vi "Marcus_3dscene.vi"() -> ()   [LabVIEW 2020]
uses:
  <vilib>/picture/3D Picture Control/Object/Create Object (name).vi
  <vilib>/picture/3D Picture Control/NI_3D Picture Control.lvlib
panel:
  in  "Dial 6":dbl(knob) scale=0.0..270.0
  in  "Dial 5":dbl(knob) scale=0.0..270.0
  in  "Dial 4":dbl(knob) scale=0.0..270.0
  in  "Dial 3":dbl(knob) scale=0.0..270.0
  in  "Dial 2":dbl(knob) scale=0.0..270.0
  in  "Dial":dbl(knob) scale=0.0..270.0
  in  "Stop":bool
  out "3D Picture":refnum<vi>(3d-picture)
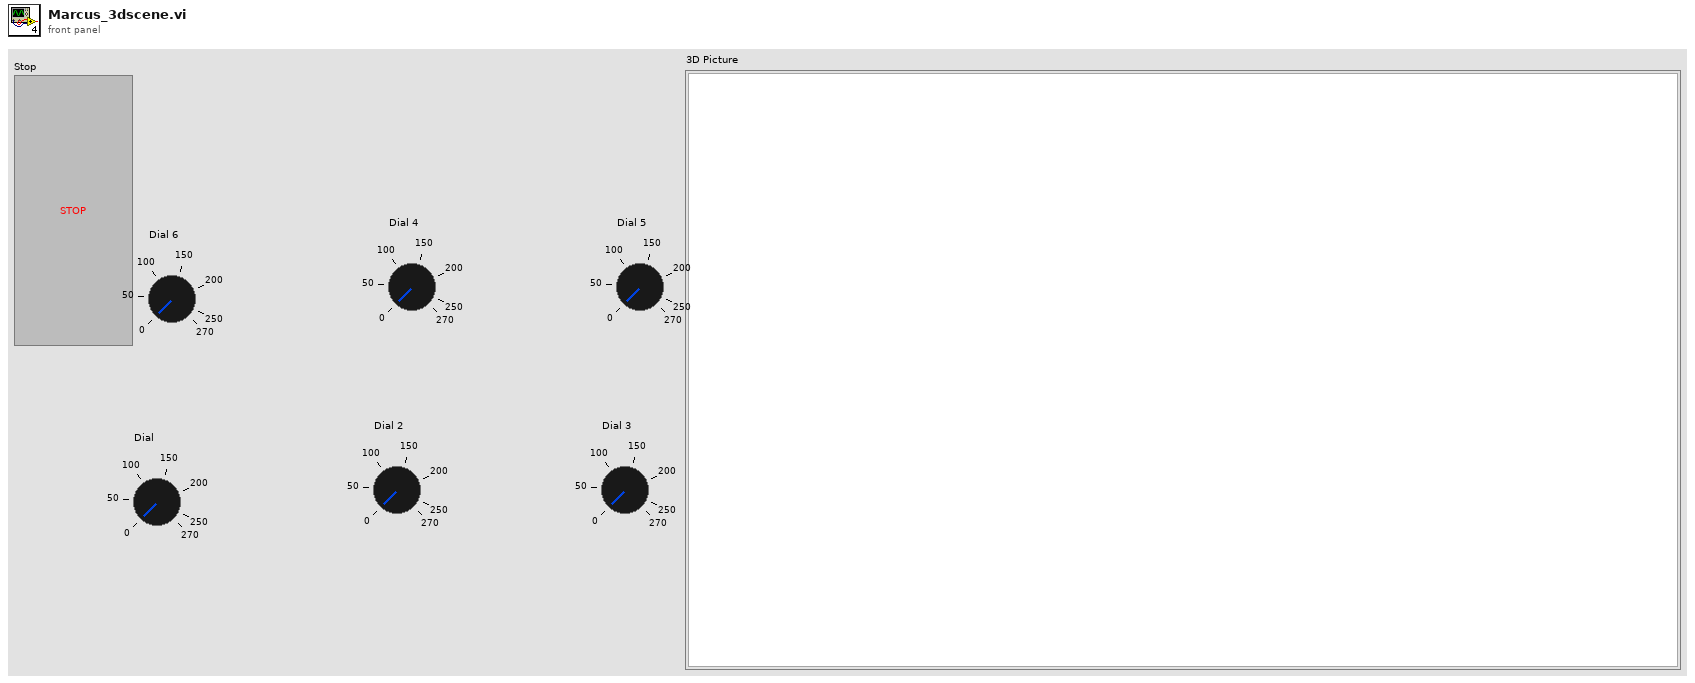
[diagram p1: front panel]
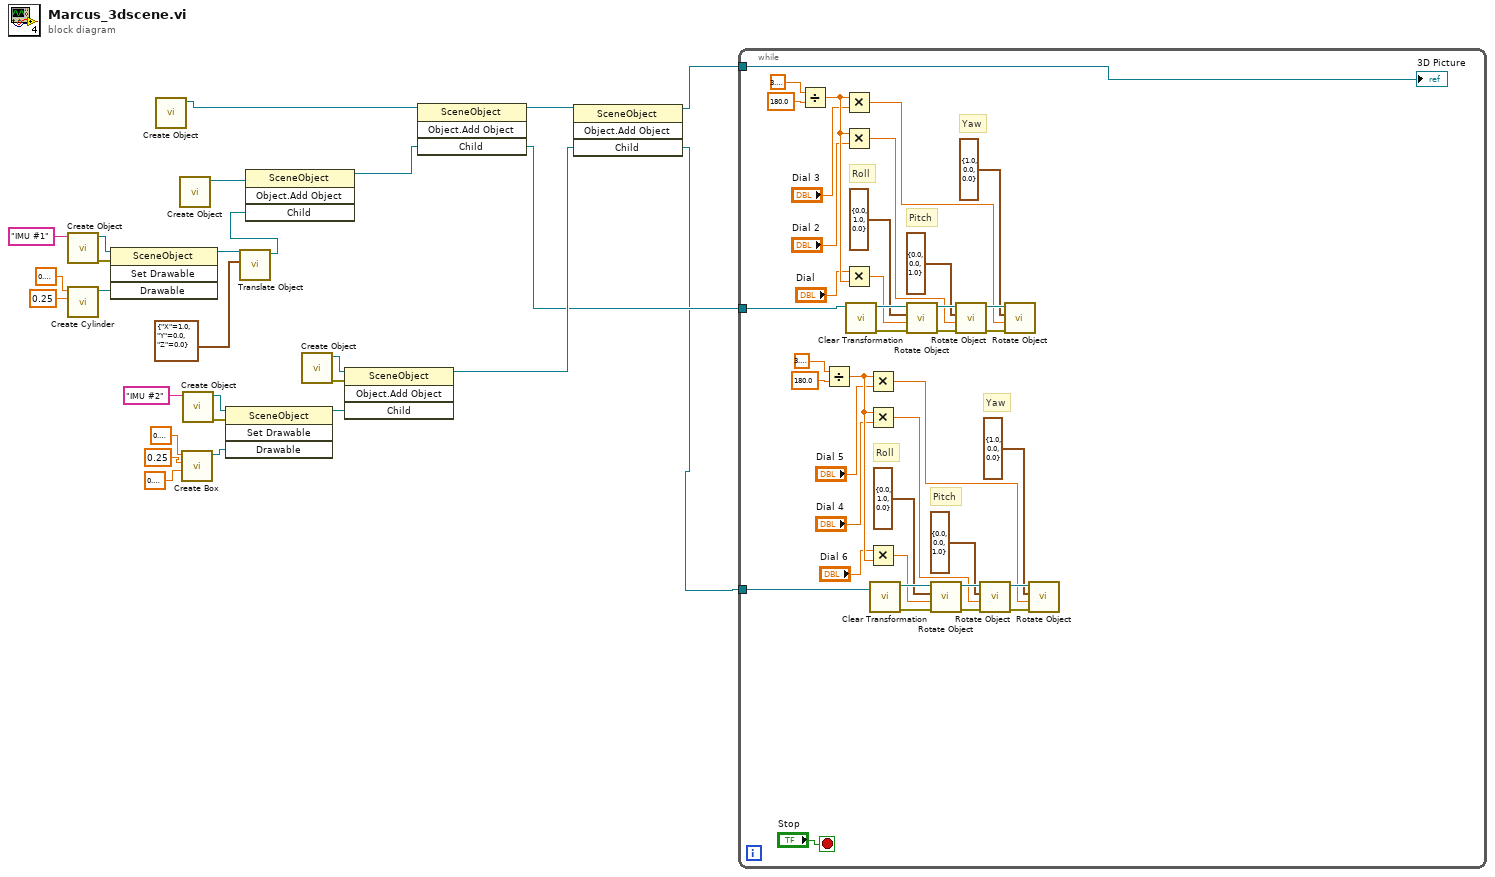
[diagram p0: block diagram]
diagram:
  n1 = call-poly <vilib>:"Create Object.vi"("Name"="IMU #1") -> ("error out"=w26:errorcluster, "Scene:New Object"=w25:refnum<vi>)  [unwired: 9 in]
  n2 = call <vilib>:"Create Cylinder.vi"("Radius"=sgl 0.25 ("Length Y"), "Height"=sgl 0.2 ("Length X")) -> ("New Cylinder Refnum"=w27:refnum<vi>)  [unwired: 8 in, 1 out]
  n3 = invoke class="SceneObject" method="Set Drawable"(reference=w25, error in=w26, "Drawable"=w27) -> (reference out=w13:refnum<vi>)  [unwired: 1 in, 3 out]
  n4 = call-poly <vilib>:"Create Object.vi"() -> ("Scene:New Object"=w11:refnum<vi>)  [unwired: 10 in, 1 out]
  n5 = call-poly <vilib>:"Create Object.vi"() -> ("Scene:New Object"=w14:refnum<vi>)  [unwired: 10 in, 1 out]
  n6 = call <vilib>:"Create Box.vi"("Length Z"=sgl 0.2, "Length Y"=sgl 0.25, "Length X"=sgl 0.2) -> ("New Box Refnum"=w1:refnum<vi>)  [unwired: 7 in, 1 out]
  n7 = call-poly <vilib>:"Create Object.vi"("Name"="IMU #2") -> ("error out"=w18:errorcluster, "Scene:New Object"=w17:refnum<vi>)  [unwired: 9 in]
  n8 = invoke class="SceneObject" method="Set Drawable"(reference=w17, error in=w18, "Drawable"=w1) -> (reference out=w21:refnum<vi>)  [unwired: 1 in, 3 out]
  n9 = call <vilib>:"Translate Object.vi"("Translation"=cluster{"X":sgl, "Y":sgl, "Z":sgl} {"X"=1.0, "Y"=0.0, "Z"=0.0}, "Scene.Object In"=w13) -> ("Scene.Object Out"=w12:refnum<vi>)  [unwired: 8 in, 1 out]
  n10 = invoke class="SceneObject" method="Object.Add Object"(reference=w14, "Child"=w12) -> (reference out=w8:refnum<vi>)  [unwired: 2 in, 3 out]
  n11 = call-poly <vilib>:"Create Object.vi"() -> ("error out"=w20:errorcluster, "Scene:New Object"=w19:refnum<vi>)  [unwired: 10 in]
  n12 = invoke class="SceneObject" method="Object.Add Object"(reference=w19, error in=w20, "Child"=w21) -> (reference out=w9:refnum<vi>)  [unwired: 1 in, 3 out]
  n13 = invoke class="SceneObject" method="Object.Add Object"(reference=w11, "Child"=w8) -> (reference out=w10:refnum<vi>, "Child"=w6:refnum<vi>)  [unwired: 2 in, 2 out]
  n14 = invoke class="SceneObject" method="Object.Add Object"(reference=w10, "Child"=w9) -> (reference out=w7:refnum<vi>, "Child"=w5:refnum<vi>)  [unwired: 2 in, 2 out]
  n15 = while {
    tunnel: w5 -> [w30]
    tunnel: w6 -> [w29]
    tunnel: w7 -> [w28]
    stop <- "Stop" stop-if-true
    # "Yaw"
    # "Pitch"
    # "Roll"
    # "Yaw"
    # "Pitch"
    # "Roll"
    n16 = Divide(x=3.141592653589793, y=180.0) -> (x/y=w52:dbl)
    n17 = Divide(x=3.141592653589793, y=180.0) -> (x/y=w34:dbl)
    n18 = Multiply(x=w52, y="Dial 3") -> (x*y=w56:dbl)
    n19 = Multiply(x=w52, y="Dial 2") -> (x*y=w53:dbl)
    n20 = Multiply(x="Dial", y=w52) -> (x*y=w54:dbl)
    n21 = call <vilib>:"Clear Transformation.vi"("Object Refnum In"=w29) -> ("error out"=w64:errorcluster, "Object Refnum Out"=w65:refnum<vi>)  [unwired: 9 in]
    n22 = Multiply(x=w34, y="Dial 5") -> (x*y=w37:dbl)
    n23 = Multiply(x=w34, y="Dial 4") -> (x*y=w35:dbl)
    n24 = Multiply(x="Dial 6", y=w34) -> (x*y=w36:dbl)
    n25 = call <vilib>:"Clear Transformation.vi"("Object Refnum In"=w30) -> ("error out"=w45:errorcluster, "Object Refnum Out"=w46:refnum<vi>)  [unwired: 9 in]
    n26 = call <vilib>:"Rotate Object.vi"("error in (no error)"=w64, "Angle"=w54, "Axis"=cluster{"X":sgl, "Y":sgl, "Z":sgl} {"X"=0.0, "Y"=1.0, "Z"=0.0}, "Scene.Object In"=w65) -> ("error out"=w66:errorcluster, "Scene.Object Out"=w67:refnum<vi>)  [unwired: 6 in]
    n27 = call <vilib>:"Rotate Object.vi"("error in (no error)"=w45, "Angle"=w36, "Axis"=cluster{"X":sgl, "Y":sgl, "Z":sgl} {"X"=0.0, "Y"=1.0, "Z"=0.0}, "Scene.Object In"=w46) -> ("error out"=w47:errorcluster, "Scene.Object Out"=w48:refnum<vi>)  [unwired: 6 in]
    n28 = call <vilib>:"Rotate Object.vi"("error in (no error)"=w66, "Angle"=w53, "Axis"=cluster{"X":sgl, "Y":sgl, "Z":sgl} {"X"=0.0, "Y"=0.0, "Z"=1.0}, "Scene.Object In"=w67) -> ("error out"=w59:errorcluster, "Scene.Object Out"=w60:refnum<vi>)  [unwired: 6 in]
    n29 = call <vilib>:"Rotate Object.vi"("error in (no error)"=w47, "Angle"=w35, "Axis"=cluster{"X":sgl, "Y":sgl, "Z":sgl} {"X"=0.0, "Y"=0.0, "Z"=1.0}, "Scene.Object In"=w48) -> ("error out"=w40:errorcluster, "Scene.Object Out"=w41:refnum<vi>)  [unwired: 6 in]
    n30 = call <vilib>:"Rotate Object.vi"("error in (no error)"=w59, "Angle"=w56, "Axis"=cluster{"X":sgl, "Y":sgl, "Z":sgl} {"X"=1.0, "Y"=0.0, "Z"=0.0}, "Scene.Object In"=w60) -> ()  [unwired: 6 in, 2 out]
    n31 = call <vilib>:"Rotate Object.vi"("error in (no error)"=w40, "Angle"=w37, "Axis"=cluster{"X":sgl, "Y":sgl, "Z":sgl} {"X"=1.0, "Y"=0.0, "Z"=0.0}, "Scene.Object In"=w41) -> ()  [unwired: 6 in, 2 out]
    "3D Picture" <- w28
  }
